vi "Post-Build Action.vi"(5 "files generated by build":path[](array[path]), 6 "top level/always included VIs":path[](array[path]), 7 "destination path":path, 8 "error in":errorcluster, 9 "target name":string, 10 "build specification name":string, 11 "project path":path) -> (0 "error out":errorcluster)   [LabVIEW 2022 SP3, in "Frequency Response.lvlib"]
uses:
  Frequency Response.lvlib
  Measurement Plugin.lvclass
  C:/Program Files/National Instruments/LabVIEW 2022/vi.lib/Plug-In SDKs/Measurements/Measurement Plugin Service/Measurement Plugin Service.lvclass
  <vilib>/Plug-In SDKs/Measurements/NI Measurement Plug-In SDK.lvlib
  C:/dev/digital-microphone/source/frequency response/Frequency Response/Advanced/Measurement Plugin.lvclass
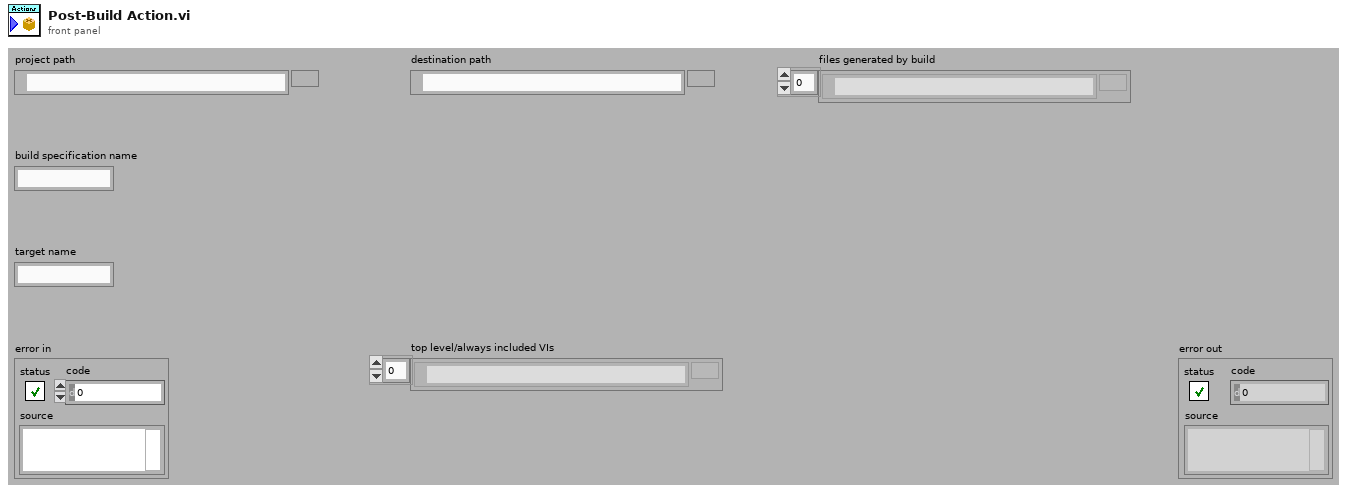
[diagram p1: front panel]
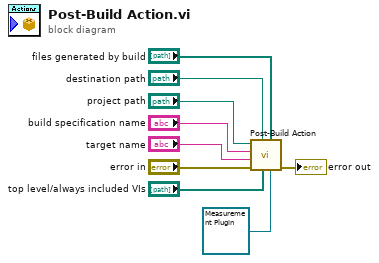
[diagram p0: block diagram]
diagram:
  n1 = call <vilib>:"Post-Build Action.vi"("measurement plugin service"=refnum<class "Measurement Plugin.lvclass"> refnum ("MeasurementLink Measurement Template.lvlib:MeasurementPlugin.lvclass"), "files generated by build"="files generated by build", "top level/always included VIs"="top level/always included VIs", "destination path"="destination path", "error in"="error in", "target name"="target name", "build specification name"="build specification name", "project path"="project path") -> ("error out"=→"error out":errorcluster)  [unwired: 3 in]
